vi "Get Pose.vi"(8 "error in (no error)":errorcluster, 11 "Rover in":refnum<class "Rover.lvclass">) -> (0 "error out":errorcluster, 2 "Pose":T1, 3 "Rover out":refnum<class "Rover.lvclass">)   [LabVIEW 2020, in "Rover.lvlib" / "Rover.lvclass"]
uses:
  Rover.lvclass
  Pose.ctl
  I2C Register.ctl
  Rover.lvclass/Rover.ctl
  <vilib>/MakerHub/LINX/Private/Local IO/LinxI2cWrite.vi
  <vilib>/MakerHub/LINX/Public/Utilities/Check Channel.vi
  <vilib>/MakerHub/LINX/Private/Local IO/Handle Errors.vi
  <vilib>/MakerHub/LINX/Private/Utilties/Generate Error.vi
  <vilib>/MakerHub/LINX/LMH-LINX.lvlib
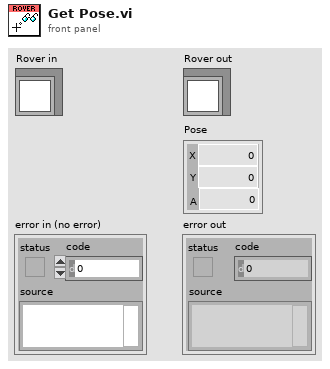
[diagram p1: front panel]
types:
  T1 = typedef "Rover.lvlib/Rover.lvclass/Pose.ctl" = cluster{"X":sgl, "Y":sgl, "A":sgl}
  T2 = typedef "Rover.lvlib/Rover.lvclass/I2C Register.ctl" = enum8{"encA", "encB", "ticksPerUnit", "width", "flags", "velP", "velI", "velD", "velMin", "velMax", "poseX", "poseY", "poseA", "cmdDrive", "cmdTurn", "velocity", "turn", "velL", "velR", "run", "outL", "outR", "outDeadband"}
  T3 = typedef "LMH-LINX.lvlib/LINX Ref.ctl" = cluster{"IO":T4, "Interface":T5, "LINX Device Config":T6}
  T4 = typedef "LMH-LINX.lvlib/Platform.ctl" = enum16{"Remote", "Local"}
  T5 = typedef "LMH-LINX.lvlib/Interface.ctl" = enum16{"Serial", "TCP"}
  T6 = typedef "LMH-LINX.lvlib/Device.lvlib/LINX Device Config.ctl" = cluster{"Interface":T5, "COM Port":refnum<visa-resource-name>, "TCP Configuration":T7, "Device Family":u8, "Device ID":u8, "Device Name":string, "TCP Ref":refnum<k5>, "Channels":T8}
  T7 = typedef "LMH-LINX.lvlib/Device.lvlib/TCP Config.ctl" = cluster{"IP Address":string, "Port":u16}
  T8 = typedef "LMH-LINX.lvlib/Channels.ctl" = cluster{"DI":u8[], "DO":u8[], "AI":u8[], "AO":u8[], "PWM":u8[], "QE":u8[], "UART":u8[], "I2C 2":u8[], "SPI":u8[], "CAN":u8[], "Servo":u8[], "AI Ref (V)":dbl, "AI Resolution (Bits)":u8, "AO Ref (V)":dbl, "AO Resolution (Bits)":u8}
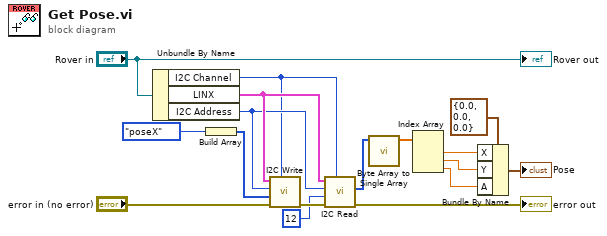
[diagram p0: block diagram]
diagram:
  n1 = Unbundle By Name("Rover in") -> ("I2C Channel"=w10:u8, "LINX"=w12:T3, "I2C Address"=w11:u8)
  n2 = Build Array(I2C_Register."poseX" ("I2C Register")) -> (w14:T2[])
  n3 = call <vilib>:"I2C Write.vi"("I2C Channel"=w10, "Error In"="error in (no error)", "Data"=w14, "I2C Slave Address (0)"=w11, "LINX Resource"=w12) -> ("Error Out"=w13:errorcluster)  [unwired: 5 in, 1 out]
  n4 = call <vilib>:"I2C Read.vi"("I2C Channel"=w10, "Error In"=w13, "Bytes To Read"=u8 12, "I2C Slave Address (0)"=w11, "LINX Resource"=w12) -> ("Error Out"=→"error out":errorcluster, "Data"=w2:u8[])  [unwired: 4 in, 1 out]
  n5 = call "Byte Array to Single Array.vi"("Byte Array"=w2) -> ("SGL Array"=w1:sgl[])  [unwired: 10 in]
  n6 = Index Array(array=w1) -> (element #1=w5:sgl, element #2=w3:sgl, element #3=w4:sgl)  [unwired: 3 in]
  n7 = Bundle By Name(cluster=T1 {"X"=0.0, "Y"=0.0, "A"=0.0} ("Pose"), "X"=w5, "Y"=w3, "A"=w4) -> (→"Pose":T1)
  "Rover out" <- "Rover in"
